vi "Release Message Transport.vi"(8 "error in (no error)":errorcluster, 11 "Message Transport in":refnum<class "Message Transport.lvclass">) -> ()   [LabVIEW 2018, in "Message Transport.lvclass"]
uses:
  Message Transport.lvclass
  Message Transport.lvclass/Message Transport.ctl
  Communication_class/Get Message Queue.vi
  Message_class/Message.lvclass
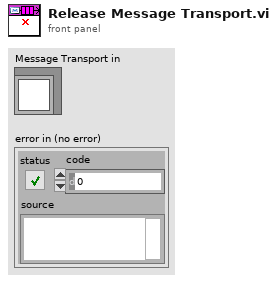
[diagram p1: front panel]
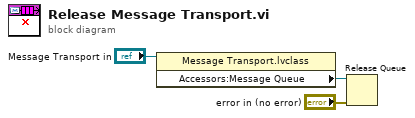
[diagram p0: block diagram]
diagram:
  n1 = property class="Message Transport.lvclass"(reference="Message Transport in") -> ("Accessors:Message Queue"=w1:refnum<queue>)  [unwired: 1 in, 2 out]
  n2 = Release Queue(queue=w1, error in (no error)="error in (no error)") -> ()  [unwired: 1 in, 3 out]
